vi "1.Main demo.vi"() -> ()   [LabVIEW 2010]
uses:
  UnderAutomation.Fanuc/UnderAutomation.Fanuc.lvlib
  C:/Users/fg/Documents/Fanuc.vi/LabVIEW_2024/UnderAutomation.Fanuc/lib/UnderAutomation.Fanuc.dll
  LabVIEW_2024/UnderAutomation.Fanuc/lib/UnderAutomation.Fanuc.dll
panel:
  out "SNPX connected":bool
  out "FTP connected":bool
  out "Telnet connected":bool
  in  "Tab Control":T1(tab)
  in  "Disconnect":bool
  in  "Test":bool
  in  "Key":string
  in  "Licensee":string
  in  "Use SNPX":bool
  in  "FTP password":string
  in  "FTP user":string
  in  "Use FTP":bool
  in  "Connect":bool
  in  "Telnet password":string
  in  "Use Telnet":bool
  in  "ConnectRoboguide":bool
  in  "RoboguideRobotPath":path caption="Path to \"Robot\" ROBOGUIDE folder that contains services.txt"
  in  "IP":string caption="Robot IP Address"
  out "License state":string
  out "Connect error":string
  in  "Unsimulate all":bool
  in  "Unsimulate":bool
  in  "Simulate":bool
  in  "Set port value":bool
  in  "Variable set value":bool
  in  "Variable new value":string caption="New value"
  in  "Variable get value":bool
  in  "Variable name":string
  out "Telnet warning":string
  out "Current position":T2
  in  "Get current position":bool
  in  "Reset alarms":bool
  in  "Get task info":bool
  in  "Task name":string caption="Task name (program without extension)"
  in  "Abort all programs":bool
  in  "Clear variable":bool
  in  "Clear Program":bool
  in  "Hold":bool
  in  "Continue":bool
  in  "Abort":bool
  in  "Pause":bool
  in  "Program name":string caption="Program name without extension"
  in  "Run":bool
  out "TelnetError":string caption="Error :"
  out "TelnetSucceed":bool caption="Succeeded"
  out "KclCommand":string caption="Last command :"
  out "TaskInfo":T3
  out "Variable value":string
  in  "port":i32(ring) items=["DIN", "DOUT", "RDO", "OPOUT", "TPOUT", "WDI", "WDO", "AIN", "AOUT", "GIN", "GOUT"]
  in  "index":i32
  in  "value":i32
  out "FTP warning":string
  out "PosReg":T4(array[cluster])
  out "StrReg":string[](array[string])
  in  "Tab Control IO state":T5(tab)
  out "UI":cluster{"Id":i32, "Name":string, "Value":bool}[](array[cluster])
  out "UO":cluster{"Id":i32, "Name":string, "Value":bool}[](array[cluster])
  out "SI":cluster{"Id":i32, "Name":string, "Value":bool}[](array[cluster])
  out "SO":cluster{"Id":i32, "Name":string, "Value":bool}[](array[cluster])
  out "DIN":cluster{"Id":i32, "Name":string, "Value":bool}[](array[cluster])
  out "DOUT":cluster{"Id":i32, "Name":string, "Value":bool}[](array[cluster])
  out "RI":cluster{"Id":i32, "Name":string, "Value":bool}[](array[cluster])
  out "RO":cluster{"Id":i32, "Name":string, "Value":bool}[](array[cluster])
  out "FLG":cluster{"Id":i32, "Name":string, "Value":bool}[](array[cluster])
  in  "Tab Control position":enum32{"World", "Joints", "User frames"}(tab)
  out "World Positions":T6(array[cluster])
  out "JointsPosition":dbl[](array[numeric])
  out "UserFramePositions":T7(array[cluster])
  in  "Get current position":bool
  in  "Get IO State":bool
  in  "Port":i32(ring) items=["DIN", "DOUT", "UI", "UO", "SI", "SO", "RI", "RO", "FLG"]
  out "Errors":T8(array[cluster])
  in  "Get all errors":bool
  in  "Get safety status":bool
  out "SafetyStatus":T9
  out "NumReg":dbl[](array[numeric])
  in  "Get numeric registers":bool
  in  "Get string registers":bool
  in  "Get position registers":bool
  out "SNPX warning":string
  in  "Tab Control snpx register":enum32{"Cartesian", "Joints"}(tab)
  in  "Cartesian position 2":T10
  in  "Write cartesian position register":bool
  in  "Joints position":dbl[](array[numeric])
  in  "Write joints position register":bool
  in  "Position register":i32
  in  "Read position register":bool
  out "Value":string
  in  "New value":string
  in  "String register":i32
  in  "Read string register":bool
  in  "Write string register":bool
  in  "Continuous read world position":bool
  out "JointsPosition":dbl[](array[numeric])
  out "Cartesian position":T11
  out "UserTool":i16
  out "error out":errorcluster
  in  "Continuous read user frame position":bool
  in  "userFrame":i32
  out "Cartesian position":T11
  out "UserTool":i16
  out "error out 2":errorcluster
  in  "Numeric register":i32
  in  "New value":sgl
  out "Value":sgl
  in  "Read numeric register":bool
  in  "Write numeric register":bool
  out "UserFrame":i16
  out "UserTool":i16
  in  "stop":bool
  out "Snpx":refnum<k24>
  out "Ftp":refnum<k24>
  out "Telnet":refnum<k24>
  out "robot":refnum<k24>
  # "UnderAutomation"
  # "https://underautomation.com/fanuc"
  # "+"
  # "LabVIEW demo app for remote control and monitoring of your Fanuc robot"
  # "Connect to robot"
  # "2. Ensure you have a trial or lifetime valid license"
  # "1. Set Fanuc robot address"
  # "This is a commercial library, you have a 30-day trial period. But you can use it forever if you buy a perpetual licence for your company (regardless of the number of robot, applications or developers)."
  # "Connect to real robot"
  # "Connect to ROBOGUIDE"
  # "If you have a license :"
  # "3. Select the services you want to connect to"
  # "Telnet"
  # "FTP"
  # "SNPX"
  # "You need option R553 \"HMI Device SNPX\" or R651 FRL"
  # "How to enable Telnet : https://underautomation.com/fanuc/documentation/enable-telnet"
  # "See : https://underautomation.com/fanuc/documentation/snpx"
  # "4. Connect to the robot"
  # "Telnet"
  # "Variables"
  # "Program execution"
  # "Task"
  # "Ports"
  # "Current position"
  # "Alarms"
  # "FTP"
  # "Current Position"
  # "IO State"
  # "Errors"
  # "Registers"
  # "Safety status"
  # "SNPX"
  # "Numeric registers"
  # "String registers"
  # "Read world position"
  # "Read user frame position"
  # "Position registers"
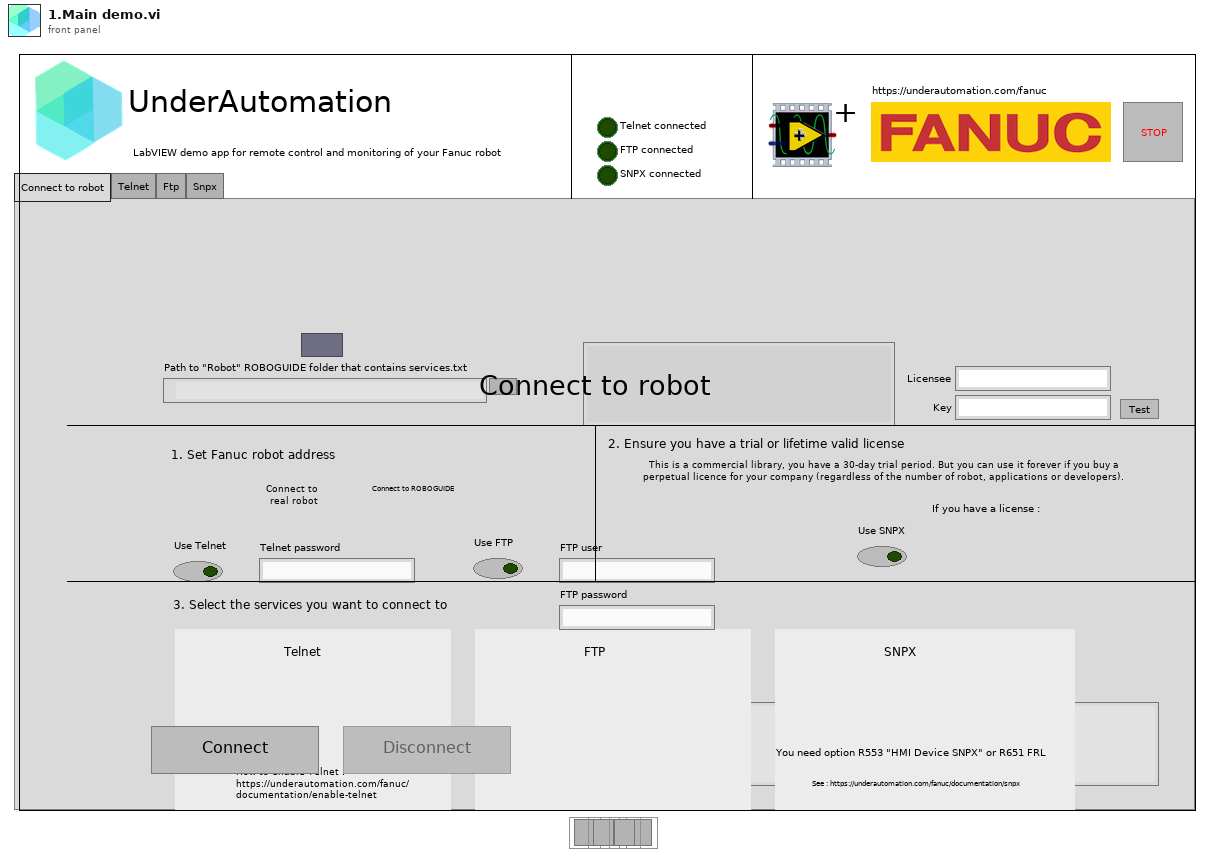
[diagram p1: front panel]
types:
  T1 = enum32{"Connect to robot", "Telnet", "Ftp", "Snpx"}
  T2 = cluster{"X":dbl, "Y":dbl, "Z":dbl, "W":dbl, "P":dbl, "R":dbl}
  T3 = cluster{"CurrentLine":i32, "RoutineName":string, "SystemTask":bool, "TaskName":string, "TaskNumber":i32, "TaskStatus":i32, "TaskStatusStr":string}
  T4 = cluster{"X":dbl, "Y":dbl, "Z":dbl, "W":dbl, "R":dbl, "P":dbl}[][]
  T5 = enum32{"UI", "UO", "SI", "SO", "DIN", "DOUT", "RI", "RO", "FLG"}
  T6 = cluster{"Tool":i32, "Cartesian position":cluster{cluster{"ArmFrontBack":i32, "ArmLeftRight":i32, "ArmUpDown":i32, "TurnAxis1":i32, "TurnAxis2":i32, "TurnAxis3":i32, "WristFlip":i32}, "X":dbl, "Y":dbl, "Z":dbl, "W":dbl, "P":dbl, "R":dbl}}[]
  T7 = cluster{"Frame":i32, "Tool":i32, "Cartesian position":cluster{cluster{"ArmFrontBack":i32, "ArmLeftRight":i32, "ArmUpDown":i32, "TurnAxis1":i32, "TurnAxis2":i32, "TurnAxis3":i32, "WristFlip":i32}, "X":dbl, "Y":dbl, "Z":dbl, "W":dbl, "P":dbl, "R":dbl}}[]
  T8 = cluster{"Id":i32, "IsReset":bool, "Text":string}[]
  T9 = cluster{"BeltBroken":bool, "ExternalEStop":bool, "FenceOpen":bool, "HandBroken":bool, "LowAirAlarm":bool, "NonTeacherEnb":bool, "OverTravel":bool, "SOPEStop":bool, "SVOFFDetect":bool, "TPDeadman":bool, "TPEnable":bool, "TPEStop":bool}
  T10 = cluster{"Configuration":cluster{"ArmFrontBack":i32, "ArmLeftRight":i32, "ArmUpDown":i32, "TurnAxis1":i32, "TurnAxis2":i32, "TurnAxis3":i32, "WristFlip":i32}, "X":dbl, "Y":dbl, "Z":dbl, "W":dbl, "P":dbl, "R":dbl}
  T11 = cluster{"Cartesian position":cluster{cluster{"ArmFrontBack":i32, "ArmLeftRight":i32, "ArmUpDown":i32, "TurnAxis1":i32, "TurnAxis2":i32, "TurnAxis3":i32, "WristFlip":i32}, "X":dbl, "Y":dbl, "Z":dbl, "W":dbl, "P":dbl, "R":dbl}, "Extension":cluster{"E1":dbl, "E2":dbl, "E3":dbl, "T4":i16, "T5":i16, "T6":i16}}
  T12 = enum8{"Enabled", "Disabled", "Disabled and Grayed Out"}
  T13 = cluster{"X":dbl, "Y":dbl, "Z":dbl, "W":dbl, "P":dbl, "R":dbl}[][]
  T14 = cluster{"Id":i32, "Values":dbl[], "UserFramePositions":cluster{"Frame":i32, "Tool":i32, "Cartesian position":cluster{cluster{"ArmFrontBack":i32, "ArmLeftRight":i32, "ArmUpDown":i32, "TurnAxis1":i32, "TurnAxis2":i32, "TurnAxis3":i32, "WristFlip":i32}, "X":dbl, "Y":dbl, "Z":dbl, "W":dbl, "P":dbl, "R":dbl}}[], "World Positions":cluster{"Tool":i32, "Cartesian position":cluster{cluster{"ArmFrontBack":i32, "ArmLeftRight":i32, "ArmUpDown":i32, "TurnAxis1":i32, "TurnAxis2":i32, "TurnAxis3":i32, "WristFlip":i32}, "X":dbl, "Y":dbl, "Z":dbl, "W":dbl, "P":dbl, "R":dbl}}[]}[]
  T15 = cluster{"Id":i32, "Name":string, "Port":i32, "Value":bool, "PortStr":string}[]
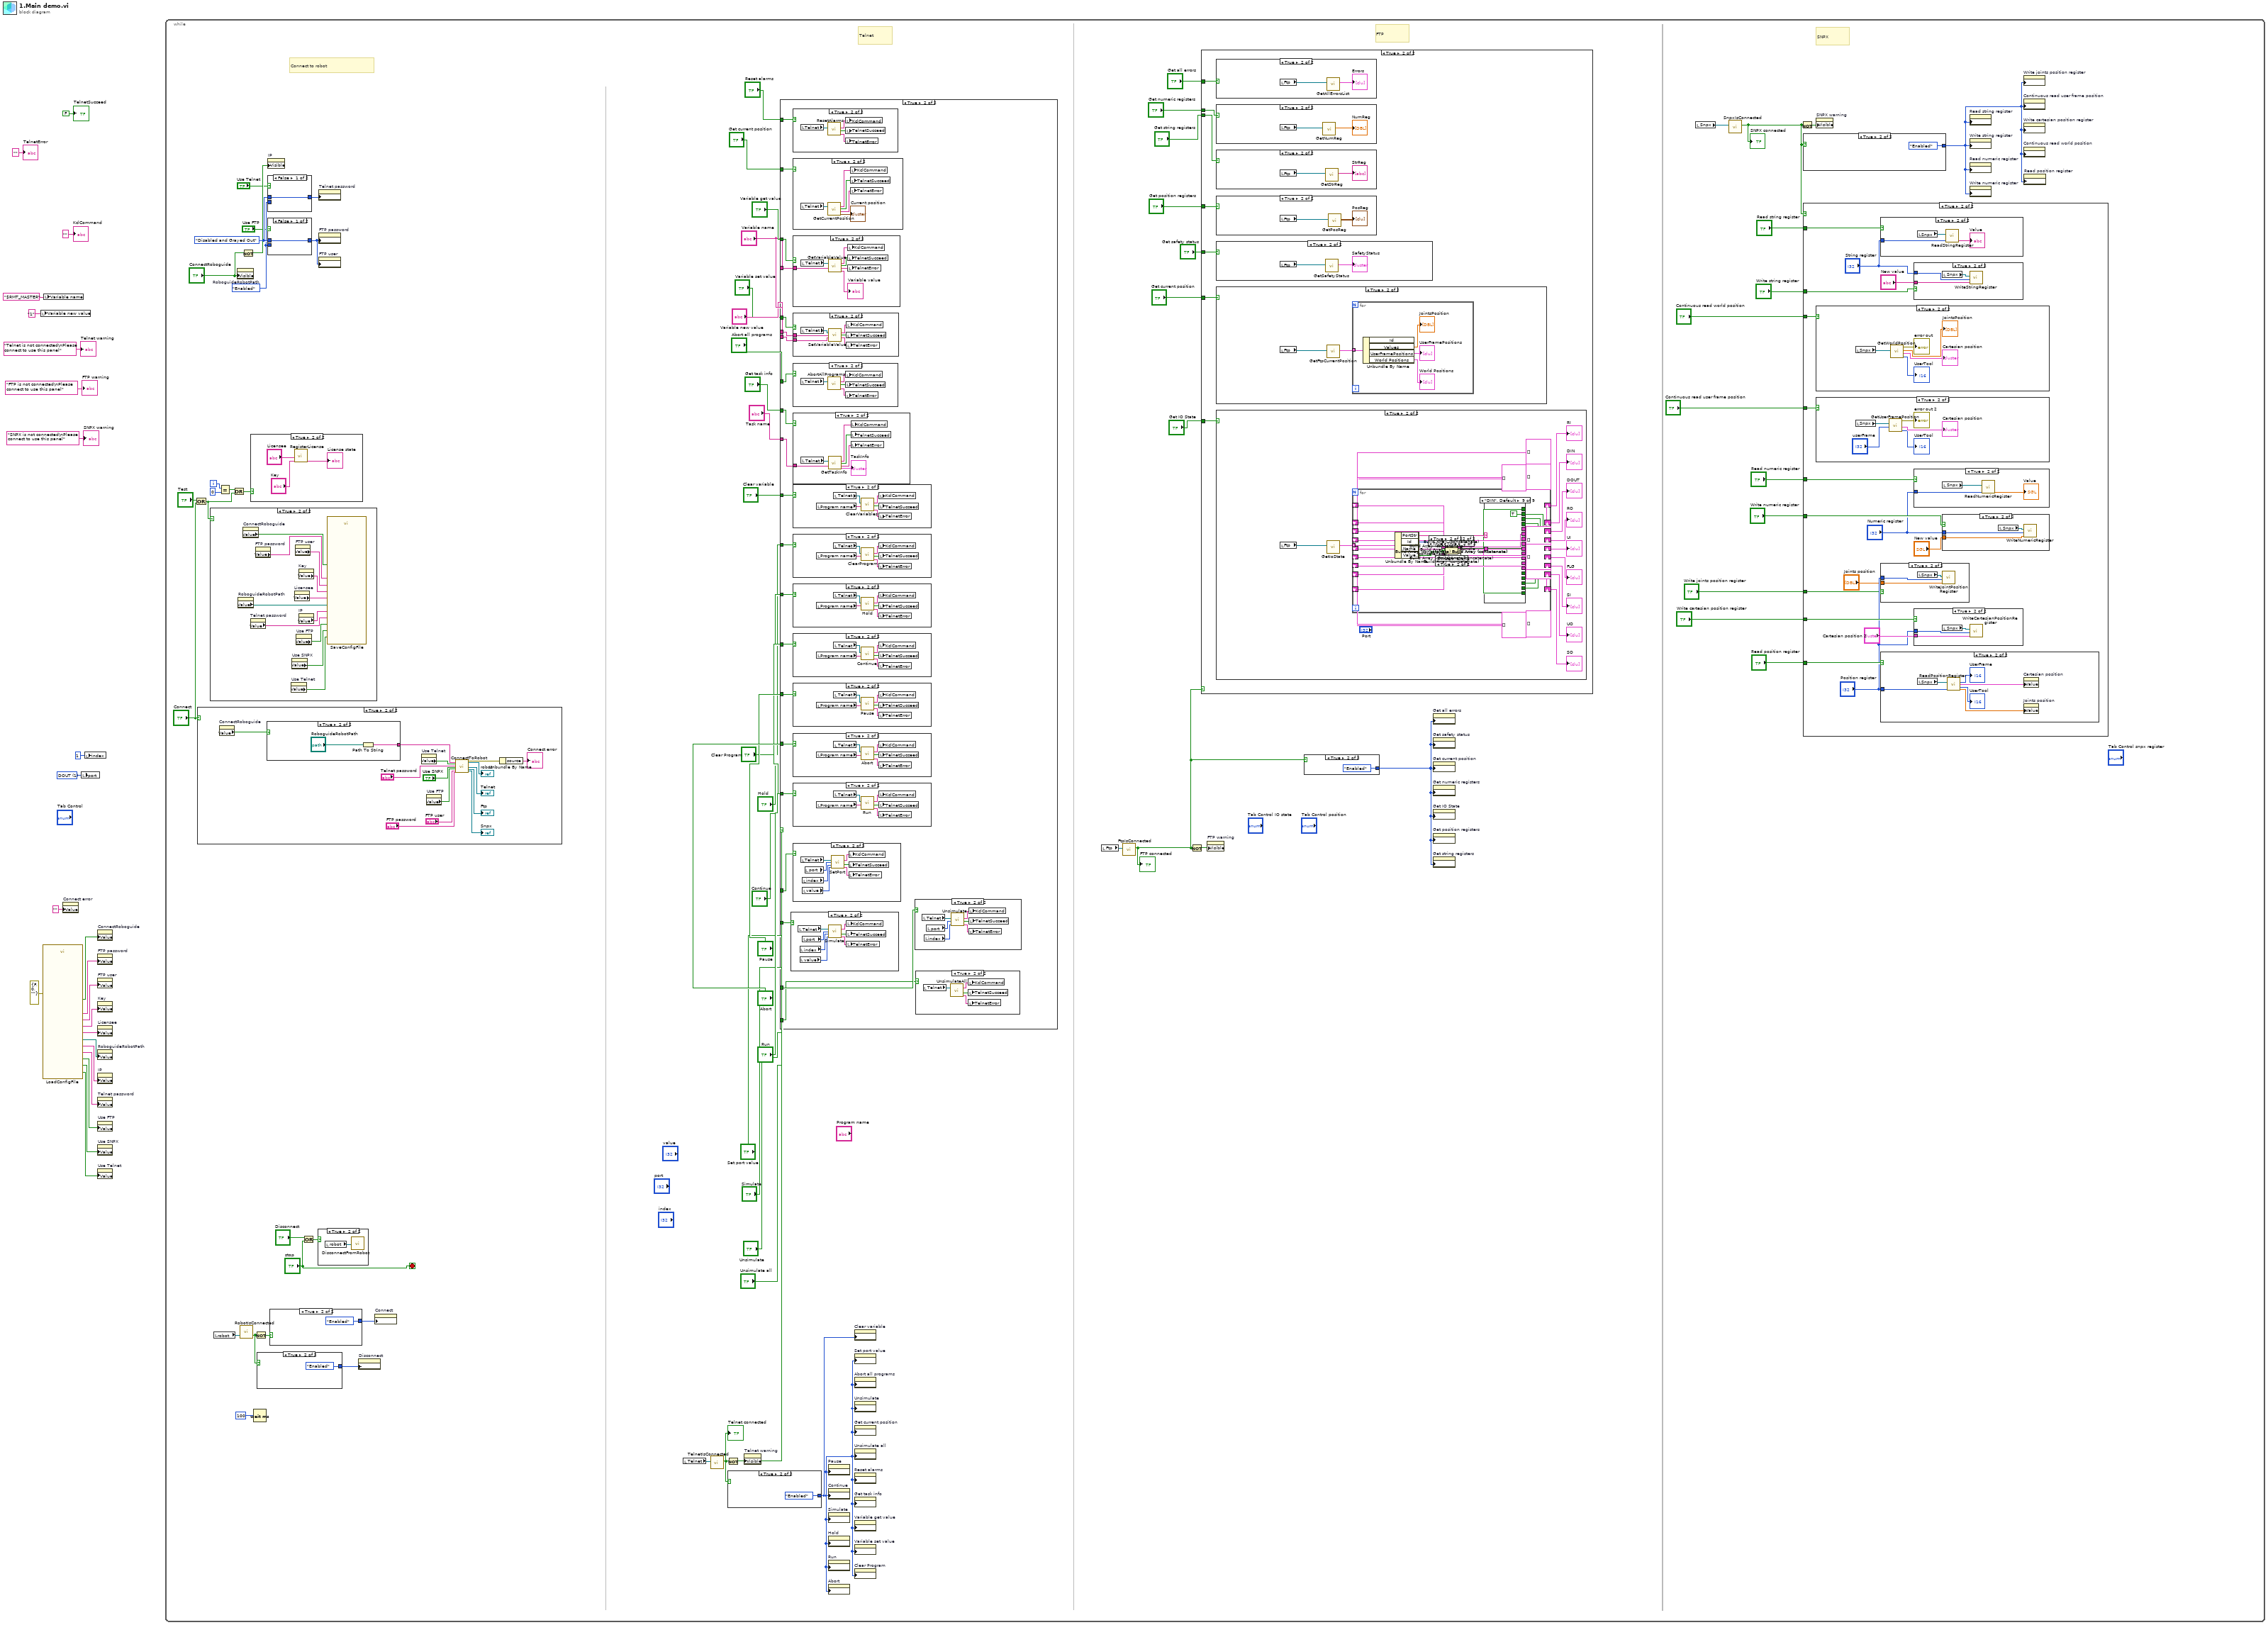
[diagram p0: block diagram]
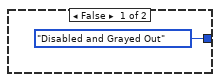
[diagram p2: hidden frame]
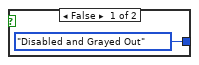
[diagram p13: hidden frame]
diagram:
  w3 = 1 items=["DIN", "DOUT", "RDO", "OPOUT", "TPOUT", "WDI", "WDO", "AIN", "AOUT", "GIN", "GOUT"] ("port")
  n1 = local write "Variable new value"("1" ("Variable new value")) -> ()
  n2 = call "LoadConfigFile.vi"("error in (no error)"=errorcluster {"status"=FALSE, "code"=0, "source"=""}) -> ("FTP password"=w20:string, "Licensee"=w12:string, "FTP user"=w19:string, "Key"=w13:string, "Use FTP"=w16:bool, "IP"=w22:string, "RoboguideRobotPath"=w18:path, "ConnectRoboguide"=w21:bool, "Use Telnet"=w14:bool, "Telnet password"=w17:string, "Use SNPX"=w15:bool)  [unwired: 15 in, 1 out]
  n3 = local write "Variable name"("$RMT_MASTER" ("Variable name")) -> ()
  n4 = property on="Connect error" class="Str"("Value"="" ("Connect error")) -> ()  [unwired: 2 in, 2 out]
  n5 = local write "port"(w3) -> ()
  n6 = local write "index"(1 ("index")) -> ()
  n7 = property on="ConnectRoboguide" class="Bool (strict)"("Value"=w21) -> ()  [unwired: 2 in, 2 out]
  n8 = property on="FTP password" class="Str"("Value"=w20) -> ()  [unwired: 2 in, 2 out]
  n9 = property on="FTP user" class="Str"("Value"=w19) -> ()  [unwired: 2 in, 2 out]
  n10 = property on="Key" class="Str"("Value"=w13) -> ()  [unwired: 2 in, 2 out]
  n11 = property on="Licensee" class="Str"("Value"=w12) -> ()  [unwired: 2 in, 2 out]
  n12 = property on="RoboguideRobotPath" class="Path"("Value"=w18) -> ()  [unwired: 2 in, 2 out]
  n13 = property on="IP" class="Str"("Value"=w22) -> ()  [unwired: 2 in, 2 out]
  n14 = property on="Telnet password" class="Str"("Value"=w17) -> ()  [unwired: 2 in, 2 out]
  n15 = property on="Use FTP" class="Bool (strict)"("Value"=w16) -> ()  [unwired: 2 in, 2 out]
  n16 = property on="Use SNPX" class="Bool (strict)"("Value"=w15) -> ()  [unwired: 2 in, 2 out]
  n17 = property on="Use Telnet" class="Bool (strict)"("Value"=w14) -> ()  [unwired: 2 in, 2 out]
  n18 = while {
    i -> [w90]
    stop <- "stop" stop-if-true
    w82 = T12."Enabled" ("Disabled")
    w83 = T12."Disabled and Grayed Out" ("Disabled")
    # "SNPX"
    # "FTP"
    # "Telnet"
    # "Connect to robot"
    n19 = Or(x="Test", y="Connect") -> (x .or. y?=w87:bool)
    n20 = case shown="True" "Connect" {
      frame False {
      }
      frame True {
        n21 = property on="ConnectRoboguide" class="Bool (strict)"() -> ("Value"=w438:bool)  [unwired: 2 in, 2 out]
        n22 = case shown="True" w438 {
          tunnel: ["IP" w440] -> w437
          frame False {
          }
          frame True {
            n23 = Path To String(path="RoboguideRobotPath") -> (string=w440:string)
          }
        }
        n24 = property on="Use Telnet" class="Bool (strict)"() -> ("Value"=w433:bool)  [unwired: 2 in, 2 out]
        n25 = property on="Use FTP" class="Bool (strict)"() -> ("Value"=w432:bool)  [unwired: 2 in, 2 out]
        n26 = call "ConnectToRobot.vi"("address"=w437, "Telnet enable"=w433, "Telnet KCL password"="Telnet password", "SNPX enable"="Use SNPX", "FTP enable"=w432, "FTP user"="FTP user", "FTP password"="FTP password") -> ("error out"=w431:errorcluster, "robot"=→"robot":refnum<k24>, "Telnet"=→"Telnet":refnum<k24>, "Ftp"=→"Ftp":refnum<k24>, "Snpx"=→"Snpx":refnum<k24>)  [unwired: 16 in]
        n27 = Unbundle By Name(w431) -> ("source"=→"Connect error":string)
      }
    }
    n28 = case shown="True" w87 {
      frame False {
      }
      frame True {
        n29 = property on="RoboguideRobotPath" class="Path"() -> ("Value"=w419:path)  [unwired: 2 in, 2 out]
        n30 = property on="ConnectRoboguide" class="Bool (strict)"() -> ("Value"=w424:bool)  [unwired: 2 in, 2 out]
        n31 = property on="Telnet password" class="Str"() -> ("Value"=w417:string)  [unwired: 2 in, 2 out]
        n32 = property on="FTP password" class="Str"() -> ("Value"=w423:string)  [unwired: 2 in, 2 out]
        n33 = property on="Use Telnet" class="Bool (strict)"() -> ("Value"=w414:bool)  [unwired: 2 in, 2 out]
        n34 = property on="Use SNPX" class="Bool (strict)"() -> ("Value"=w415:bool)  [unwired: 2 in, 2 out]
        n35 = property on="Licensee" class="Str"() -> ("Value"=w420:string)  [unwired: 2 in, 2 out]
        n36 = property on="FTP user" class="Str"() -> ("Value"=w422:string)  [unwired: 2 in, 2 out]
        n37 = property on="Use FTP" class="Bool (strict)"() -> ("Value"=w416:bool)  [unwired: 2 in, 2 out]
        n38 = property on="Key" class="Str"() -> ("Value"=w421:string)  [unwired: 2 in, 2 out]
        n39 = property on="IP" class="Str"() -> ("Value"=w418:string)  [unwired: 2 in, 2 out]
        n40 = call "SaveConfigFile.vi"("IP"=w418, "RoboguideRobotPath"=w419, "ConnectRoboguide"=w424, "Use Telnet"=w414, "Telnet password"=w417, "Use FTP"=w416, "FTP user"=w422, "FTP password"=w423, "Use SNPX"=w415, "Licensee"=w420, "Key"=w421) -> ()  [unwired: 17 in]
      }
    }
    n41 = local read "robot"() -> (w57:refnum<k24>)
    n42 = Equal?(x=w90, y=0) -> (x = y?=w88:bool)
    n43 = Or(x=w88, y=w87) -> (x .or. y?=w86:bool)
    n44 = property on="RoboguideRobotPath" class="Path"("Visible"="ConnectRoboguide") -> ()  [unwired: 2 in, 2 out]
    n45 = call "RobotIsConnected.vi"("robot"=w57) -> ("Connected"=w55:bool)  [unwired: 1 in, 1 out]
    n46 = Not(x="ConnectRoboguide") -> (.not. x?=w94:bool)
    n47 = case shown="True" w86 {
      frame False {
      }
      frame True {
        n48 = call "RegisterLicense.vi"("key"="Key", "licensee"="Licensee") -> ("status"=→"License state":string)  [unwired: 7 in, 2 out]
      }
    }
    n49 = Wait (ms)(milliseconds to wait=u32 100) -> ()  [unwired: 1 out]
    n50 = Not(x=w55) -> (.not. x?=w56:bool)
    n51 = case shown="True" w55 {
      tunnel: [T12."Disabled and Grayed Out" ("Disabled") T12."Enabled" ("Disabled")] -> w54
      frame False {
      }
      frame True {
      }
    }
    n52 = property on="IP" class="Str"("Visible"=w94) -> ()  [unwired: 2 in, 2 out]
    n53 = case shown="False" "Use Telnet" {
      tunnel: w82 -> [_ w410]
      tunnel: [w409 w410] -> w84
      tunnel: w83 -> [w409 _]
      frame False {
      }
      frame True {
      }
    }
    n54 = case shown="False" "Use FTP" {
      tunnel: w82 -> [_ w408]
      tunnel: [w407 w408] -> w80
      tunnel: w83 -> [w407 _]
      frame False {
      }
      frame True {
      }
    }
    n55 = case shown="True" w56 {
      tunnel: [T12."Disabled and Grayed Out" ("Disabled") T12."Enabled" ("Disabled")] -> w53
      frame False {
      }
      frame True {
      }
    }
    n56 = Or(x="Disconnect", y="stop") -> (x .or. y?=w59:bool)
    n57 = case shown="True" w59 {
      frame False {
      }
      frame True {
        n58 = local read "robot"() -> (w293:refnum<k24>)
        n59 = call "DisconnectFromRobot.vi"("robot"=w293) -> ()  [unwired: 26 in, 1 out]
      }
    }
    n60 = property on="Telnet password" class="Str"("DisabledEnum"=w84) -> ()  [unwired: 2 in, 2 out]
    n61 = property on="FTP password" class="Str"("DisabledEnum"=w80) -> ()  [unwired: 2 in, 2 out]
    n62 = property on="FTP user" class="Str"("DisabledEnum"=w80) -> ()  [unwired: 2 in, 2 out]
    n63 = property on="Disconnect" class="Bool"("DisabledEnum"=w54) -> ()  [unwired: 2 in, 2 out]
    n64 = property on="Connect" class="Bool"("DisabledEnum"=w53) -> ()  [unwired: 2 in, 2 out]
    n65 = local read "Telnet"() -> (w79:refnum<k24>)
    n66 = call "TelnetIsConnected.vi"("Telnet"=w79) -> ("Connected"=w77:bool)  [unwired: 9 in, 1 out]
    "Telnet connected" <- w77
    n67 = Not(x=w77) -> (.not. x?=w76:bool)
    n68 = case shown="True" w77 {
      tunnel: [T12."Disabled and Grayed Out" ("Disabled") T12."Enabled" ("Disabled")] -> w48
      frame False {
      }
      frame True {
      }
    }
    n69 = property on="Telnet warning" class="Str"("Visible"=w76) -> ()  [unwired: 2 in, 2 out]
    n70 = case shown="True" w77 {
      tunnel: "Run" -> [_ w316]
      tunnel: "Abort" -> [_ w315]
      tunnel: "Pause" -> [_ w314]
      tunnel: "Continue" -> [_ w313]
      tunnel: "Hold" -> [_ w312]
      tunnel: "Clear variable" -> [_ w311]
      tunnel: "Clear Program" -> [_ w310]
      tunnel: "Abort all programs" -> [_ w309]
      tunnel: "Task name" -> [_ w308]
      tunnel: "Get task info" -> [_ w307]
      tunnel: "Reset alarms" -> [_ w306]
      tunnel: "Get current position" -> [_ w305]
      tunnel: "Variable get value" -> [_ w304]
      tunnel: "Variable name" -> [_ w303]
      tunnel: "Variable name" -> [_ w302]
      tunnel: "Variable new value" -> [_ w301]
      tunnel: "Variable set value" -> [_ w300]
      tunnel: "Set port value" -> [_ w299]
      tunnel: "Simulate" -> [_ w298]
      tunnel: "Unsimulate" -> [_ w297]
      tunnel: "Unsimulate all" -> [_ w296]
      frame False {
      }
      frame True {
        n71 = case shown="True" w298 {
          frame False {
          }
          frame True {
            n72 = local read "Telnet"() -> (w330:refnum<k24>)
            n73 = local read "index"() -> (w327:i32)
            n74 = local read "value"() -> (w329:i32)
            n75 = local read "port"() -> (w328:i32)
            n76 = call "Simulate.vi"("Telnet"=w330, "port"=w328, "index"=w327, "value"=w329) -> ("KclCommand"=w333:string, "Succeed"=w332:bool, "ErrorText"=w331:string)  [unwired: 8 in, 1 out]
            n77 = local write "KclCommand"(w333) -> ()
            n78 = local write "TelnetSucceed"(w332) -> ()
            n79 = local write "TelnetError"(w331) -> ()
          }
        }
        n80 = case shown="True" w306 {
          frame False {
          }
          frame True {
            n81 = local read "Telnet"() -> (w361:refnum<k24>)
            n82 = call "ResetAlarms.vi"("Telnet"=w361) -> ("ErrorText"=w359:string, "Succeed"=w360:bool, "KclCommand"=w358:string)  [unwired: 7 in, 1 out]
            n83 = local write "KclCommand"(w358) -> ()
            n84 = local write "TelnetSucceed"(w360) -> ()
            n85 = local write "TelnetError"(w359) -> ()
          }
        }
        n86 = case shown="True" w305 {
          frame False {
          }
          frame True {
            n87 = local read "Telnet"() -> (w357:refnum<k24>)
            n88 = call "GetCurrentPosition.vi"("Telnet"=w357) -> ("KclCommand"=w355:string, "Succeed"=w354:bool, "ErrorText"=w353:string, "Position"=→"Current position":T2)  [unwired: 10 in, 1 out]
            n89 = local write "KclCommand"(w355) -> ()
            n90 = local write "TelnetSucceed"(w354) -> ()
            n91 = local write "TelnetError"(w353) -> ()
          }
        }
        n92 = case shown="True" w304 {
          tunnel: w303 -> [_ w351]
          frame False {
          }
          frame True {
            n93 = local read "Telnet"() -> (w352:refnum<k24>)
            n94 = call "GetVariableValue.vi"("Telnet"=w352, "name"=w351) -> ("KclCommand"=w347:string, "Succeed"=w348:bool, "ErrorText"=w349:string, "RawValue"=→"Variable value":string)  [unwired: 9 in, 1 out]
            n95 = local write "KclCommand"(w347) -> ()
            n96 = local write "TelnetSucceed"(w348) -> ()
            n97 = local write "TelnetError"(w349) -> ()
          }
        }
        n98 = case shown="True" w300 {
          tunnel: w302 -> [_ w345]
          tunnel: w301 -> [_ w344]
          frame False {
          }
          frame True {
            n99 = local read "Telnet"() -> (w346:refnum<k24>)
            n100 = call "SetVariableValue.vi"("Telnet"=w346, "value"=w344, "name"=w345) -> ("KclCommand"=w343:string, "Succeed"=w342:bool, "ErrorText"=w341:string)  [unwired: 9 in, 1 out]
            n101 = local write "KclCommand"(w343) -> ()
            n102 = local write "TelnetSucceed"(w342) -> ()
            n103 = local write "TelnetError"(w341) -> ()
          }
        }
        n104 = case shown="True" w309 {
          frame False {
          }
          frame True {
            n105 = local read "Telnet"() -> (w368:refnum<k24>)
            n106 = call "AbortAllPrograms.vi"("Telnet"=w368) -> ("ErrorText"=w369:string, "Succeed"=w370:bool, "KclCommand"=w371:string)  [unwired: 7 in, 1 out]
            n107 = local write "KclCommand"(w371) -> ()
            n108 = local write "TelnetSucceed"(w370) -> ()
            n109 = local write "TelnetError"(w369) -> ()
          }
        }
        n110 = case shown="True" w307 {
          tunnel: w308 -> [_ w366]
          frame False {
          }
          frame True {
            n111 = local read "Telnet"() -> (w367:refnum<k24>)
            n112 = call "GetTaskInfo.vi"("Telnet"=w367, "task"=w366) -> ("KclCommand"=w364:string, "Succeed"=w363:bool, "ErrorText"=w362:string, "TaskInfo"=→"TaskInfo":T3)  [unwired: 9 in, 1 out]
            n113 = local write "KclCommand"(w364) -> ()
            n114 = local write "TelnetSucceed"(w363) -> ()
            n115 = local write "TelnetError"(w362) -> ()
          }
        }
        n116 = case shown="True" w311 {
          frame False {
          }
          frame True {
            n117 = local read "Program name"() -> (w372:string)
            n118 = local read "Telnet"() -> (w373:refnum<k24>)
            n119 = call "ClearVariables.vi"("program"=w372, "Telnet"=w373) -> ("ErrorText"=w374:string, "Succeed"=w375:bool, "KclCommand"=w376:string)  [unwired: 6 in, 1 out]
            n120 = local write "KclCommand"(w376) -> ()
            n121 = local write "TelnetSucceed"(w375) -> ()
            n122 = local write "TelnetError"(w374) -> ()
          }
        }
        n123 = case shown="True" w310 {
          frame False {
          }
          frame True {
            n124 = local read "Program name"() -> (w377:string)
            n125 = local read "Telnet"() -> (w378:refnum<k24>)
            n126 = call "ClearProgram.vi"("program"=w377, "Telnet"=w378) -> ("ErrorText"=w379:string, "Succeed"=w380:bool, "KclCommand"=w381:string)  [unwired: 6 in, 1 out]
            n127 = local write "KclCommand"(w381) -> ()
            n128 = local write "TelnetSucceed"(w380) -> ()
            n129 = local write "TelnetError"(w379) -> ()
          }
        }
        n130 = case shown="True" w312 {
          frame False {
          }
          frame True {
            n131 = local read "Program name"() -> (w382:string)
            n132 = local read "Telnet"() -> (w383:refnum<k24>)
            n133 = call "Hold.vi"("program"=w382, "Telnet"=w383) -> ("ErrorText"=w384:string, "Succeed"=w385:bool, "KclCommand"=w386:string)  [unwired: 6 in, 1 out]
            n134 = local write "KclCommand"(w386) -> ()
            n135 = local write "TelnetSucceed"(w385) -> ()
            n136 = local write "TelnetError"(w384) -> ()
          }
        }
        n137 = case shown="True" w313 {
          frame False {
          }
          frame True {
            n138 = local read "Program name"() -> (w387:string)
            n139 = local read "Telnet"() -> (w388:refnum<k24>)
            n140 = call "Continue.vi"("program"=w387, "Telnet"=w388) -> ("ErrorText"=w389:string, "Succeed"=w390:bool, "KclCommand"=w391:string)  [unwired: 6 in, 1 out]
            n141 = local write "KclCommand"(w391) -> ()
            n142 = local write "TelnetSucceed"(w390) -> ()
            n143 = local write "TelnetError"(w389) -> ()
          }
        }
        n144 = case shown="True" w314 {
          frame False {
          }
          frame True {
            n145 = local read "Program name"() -> (w392:string)
            n146 = local read "Telnet"() -> (w393:refnum<k24>)
            n147 = call "Pause.vi"("program"=w392, "Telnet"=w393) -> ("ErrorText"=w394:string, "Succeed"=w395:bool, "KclCommand"=w396:string)  [unwired: 6 in, 1 out]
            n148 = local write "KclCommand"(w396) -> ()
            n149 = local write "TelnetSucceed"(w395) -> ()
            n150 = local write "TelnetError"(w394) -> ()
          }
        }
        n151 = case shown="True" w315 {
          frame False {
          }
          frame True {
            n152 = local read "Program name"() -> (w397:string)
            n153 = local read "Telnet"() -> (w398:refnum<k24>)
            n154 = call "Abort.vi"("program"=w397, "Telnet"=w398) -> ("ErrorText"=w399:string, "Succeed"=w400:bool, "KclCommand"=w401:string)  [unwired: 6 in, 1 out]
            n155 = local write "KclCommand"(w401) -> ()
            n156 = local write "TelnetSucceed"(w400) -> ()
            n157 = local write "TelnetError"(w399) -> ()
          }
        }
        n158 = case shown="True" w316 {
          frame False {
          }
          frame True {
            n159 = local read "Program name"() -> (w402:string)
            n160 = local read "Telnet"() -> (w403:refnum<k24>)
            n161 = call "Run.vi"("program"=w402, "Telnet"=w403) -> ("ErrorText"=w404:string, "Succeed"=w405:bool, "KclCommand"=w406:string)  [unwired: 6 in, 1 out]
            n162 = local write "KclCommand"(w406) -> ()
            n163 = local write "TelnetSucceed"(w405) -> ()
            n164 = local write "TelnetError"(w404) -> ()
          }
        }
        n165 = case shown="True" w299 {
          frame False {
          }
          frame True {
            n166 = local read "Telnet"() -> (w337:refnum<k24>)
            n167 = local read "index"() -> (w334:i32)
            n168 = local read "value"() -> (w336:i32)
            n169 = local read "port"() -> (w335:i32)
            n170 = call "SetPort.vi"("Telnet"=w337, "port"=w335, "index"=w334, "value"=w336) -> ("KclCommand"=w340:string, "Succeed"=w339:bool, "ErrorText"=w338:string)  [unwired: 8 in, 1 out]
            n171 = local write "KclCommand"(w340) -> ()
            n172 = local write "TelnetSucceed"(w339) -> ()
            n173 = local write "TelnetError"(w338) -> ()
          }
        }
        n174 = case shown="True" w297 {
          frame False {
          }
          frame True {
            n175 = local read "Telnet"() -> (w323:refnum<k24>)
            n176 = local read "index"() -> (w321:i32)
            n177 = local read "port"() -> (w322:i32)
            n178 = call "Unsimulate.vi"("index"=w321, "port"=w322, "Telnet"=w323) -> ("ErrorText"=w324:string, "Succeed"=w325:bool, "KclCommand"=w326:string)  [unwired: 5 in, 1 out]
            n179 = local write "KclCommand"(w326) -> ()
            n180 = local write "TelnetSucceed"(w325) -> ()
            n181 = local write "TelnetError"(w324) -> ()
          }
        }
        n182 = case shown="True" w296 {
          frame False {
          }
          frame True {
            n183 = local read "Telnet"() -> (w317:refnum<k24>)
            n184 = call "UnsimulateAll.vi"("Telnet"=w317) -> ("KclCommand"=w320:string, "Succeed"=w319:bool, "ErrorText"=w318:string)  [unwired: 11 in, 1 out]
            n185 = local write "KclCommand"(w320) -> ()
            n186 = local write "TelnetSucceed"(w319) -> ()
            n187 = local write "TelnetError"(w318) -> ()
          }
        }
      }
    }
    n188 = property on="Pause" class="Bool"("DisabledEnum"=w48) -> ()  [unwired: 2 in, 2 out]
    n189 = property on="Continue" class="Bool"("DisabledEnum"=w48) -> ()  [unwired: 2 in, 2 out]
    n190 = property on="Simulate" class="Bool"("DisabledEnum"=w48) -> ()  [unwired: 2 in, 2 out]
    n191 = property on="Hold" class="Bool"("DisabledEnum"=w48) -> ()  [unwired: 2 in, 2 out]
    n192 = property on="Run" class="Bool"("DisabledEnum"=w48) -> ()  [unwired: 2 in, 2 out]
    n193 = property on="Abort" class="Bool"("DisabledEnum"=w48) -> ()  [unwired: 2 in, 2 out]
    n194 = property on="Clear variable" class="Bool"("DisabledEnum"=w48) -> ()  [unwired: 2 in, 2 out]
    n195 = property on="Set port value" class="Bool"("DisabledEnum"=w48) -> ()  [unwired: 2 in, 2 out]
    n196 = property on="Abort all programs" class="Bool"("DisabledEnum"=w48) -> ()  [unwired: 2 in, 2 out]
    n197 = property on="Unsimulate" class="Bool"("DisabledEnum"=w48) -> ()  [unwired: 2 in, 2 out]
    n198 = property on="Get current position" class="Bool"("DisabledEnum"=w48) -> ()  [unwired: 2 in, 2 out]
    n199 = property on="Unsimulate all" class="Bool"("DisabledEnum"=w48) -> ()  [unwired: 2 in, 2 out]
    n200 = property on="Reset alarms" class="Bool"("DisabledEnum"=w48) -> ()  [unwired: 2 in, 2 out]
    n201 = property on="Get task info" class="Bool"("DisabledEnum"=w48) -> ()  [unwired: 2 in, 2 out]
    n202 = property on="Variable get value" class="Bool"("DisabledEnum"=w48) -> ()  [unwired: 2 in, 2 out]
    n203 = property on="Variable set value" class="Bool"("DisabledEnum"=w48) -> ()  [unwired: 2 in, 2 out]
    n204 = property on="Clear Program" class="Bool"("DisabledEnum"=w48) -> ()  [unwired: 2 in, 2 out]
    n205 = local read "Ftp"() -> (w47:refnum<k24>)
    n206 = call "FtpIsConnected.vi"("Ftp"=w47) -> ("Connected"=w38:bool)  [unwired: 9 in, 1 out]
    "FTP connected" <- w38
    n207 = Not(x=w38) -> (.not. x?=w39:bool)
    n208 = case shown="True" w38 {
      tunnel: "Get current position" -> [_ w156]
      tunnel: "Get IO State" -> [_ w155]
      tunnel: "Get all errors" -> [_ w154]
      tunnel: "Get safety status" -> [_ w153]
      tunnel: "Get numeric registers" -> [_ w152]
      tunnel: "Get string registers" -> [_ w151]
      tunnel: "Get position registers" -> [_ w150]
      frame False {
      }
      frame True {
        n209 = case shown="True" w154 {
          frame False {
          }
          frame True {
            n210 = local read "Ftp"() -> (w166:refnum<k24>)
            n211 = call "GetAllErrorsList.vi"("Ftp"=w166) -> ("Errors"=→"Errors":T8)  [unwired: 9 in, 1 out]
          }
        }
        n212 = case shown="True" w152 {
          frame False {
          }
          frame True {
            n213 = local read "Ftp"() -> (w162:refnum<k24>)
            n214 = call "GetNumReg.vi"("Ftp"=w162) -> ("NumReg"=→"NumReg":dbl[])  [unwired: 9 in, 1 out]
          }
        }
        n215 = case shown="True" w151 {
          frame False {
          }
          frame True {
            n216 = local read "Ftp"() -> (w160:refnum<k24>)
            n217 = call "GetStrReg.vi"("Ftp"=w160) -> ("StrReg"=→"StrReg":string[])  [unwired: 9 in, 1 out]
          }
        }
        n218 = case shown="True" w150 {
          frame False {
          }
          frame True {
            n219 = local read "Ftp"() -> (w158:refnum<k24>)
            n220 = call "GetPosReg.vi"("Ftp"=w158) -> ("PosReg"=→"PosReg":T13)  [unwired: 9 in, 1 out]
          }
        }
        n221 = case shown="True" w153 {
          frame False {
          }
          frame True {
            n222 = local read "Ftp"() -> (w164:refnum<k24>)
            n223 = call "GetSafetyStatus.vi"("Ftp"=w164) -> ("SafetyStatus"=→"SafetyStatus":T9)  [unwired: 9 in, 1 out]
          }
        }
        n224 = case shown="True" w156 {
          frame False {
          }
          frame True {
            n225 = local read "Ftp"() -> (w284:refnum<k24>)
            n226 = call "GetFtpCurrentPosition.vi"("Ftp"=w284) -> ("Current position"=w283:T14)  [unwired: 9 in, 1 out]
            n227 = for {
              tunnel: w283 -> [w287] mode=indexing
              n228 = Unbundle By Name(w287) -> ("Values"=→"JointsPosition":dbl[], "UserFramePositions"=→"UserFramePositions":T7, "World Positions"=→"World Positions":T6)  [unwired: 1 out]
            }
          }
        }
        n229 = case shown="True" w155 {
          frame False {
          }
          frame True {
            n230 = local read "Ftp"() -> (w186:refnum<k24>)
            n231 = call "GetIoState.vi"("Ftp"=w186) -> ("IO States"=w185:T15)  [unwired: 9 in, 1 out]
            n232 = for {
              tunnel: w185 -> [w228] mode=indexing
              shift-right: [w203] -> w184
              shift-left: cluster{"Id":i32, "Name":string, "Value":bool}[] [] ("Array") -> [w204]
              shift-right: [w201] -> w183
              shift-left: cluster{"Id":i32, "Name":string, "Value":bool}[] [] ("Array") -> [w202]
              shift-right: [w199] -> w176
              shift-left: cluster{"Id":i32, "Name":string, "Value":bool}[] [] ("Array") -> [w200]
              shift-right: [w197] -> w182
              shift-left: cluster{"Id":i32, "Name":string, "Value":bool}[] [] ("Array") -> [w198]
              shift-right: [w195] -> w181
              shift-left: cluster{"Id":i32, "Name":string, "Value":bool}[] [] ("Array") -> [w196]
              shift-right: [w193] -> w180
              shift-left: cluster{"Id":i32, "Name":string, "Value":bool}[] [] ("Array") -> [w194]
              shift-right: [w191] -> w179
              shift-left: cluster{"Id":i32, "Name":string, "Value":bool}[] [] ("Array") -> [w192]
              shift-right: [w189] -> w178
              shift-left: cluster{"Id":i32, "Name":string, "Value":bool}[] [] ("Array") -> [w190]
              shift-right: [w187] -> w177
              shift-left: cluster{"Id":i32, "Name":string, "Value":bool}[] [] ("Array") -> [w188]
              n233 = Unbundle By Name(w228) -> ("PortStr"=w216:string, "Id"=w227:i32, "Name"=w226:string, "Value"=w225:bool)
              n234 = Bundle("Id"=w227, "Name"=w226, "Value"=w225) -> (w223:cluster{"Id":i32, "Name":string, "Value":bool})  [unwired: 1 in]
              n235 = case shown="\"DIN\", Default" w216 {
                tunnel: [_ _ _ _ _ _ _ w280 _] -> w224
                tunnel: w223 -> [w266 w268 w270 w272 w274 w276 w278 w280 w282]
                tunnel: [_ _ _ _ _ _ w278 _ _] -> w222
                tunnel: [_ _ _ _ _ _ _ _ w282] -> w214
                tunnel: [w266 _ _ _ _ _ _ _ _] -> w221
                tunnel: [_ w268 _ _ _ _ _ _ _] -> w220
                tunnel: [_ _ w270 _ _ _ _ _ _] -> w219
                tunnel: [_ _ _ w272 _ _ _ _ _] -> w218
                tunnel: [_ _ _ _ w274 _ _ _ _] -> w217
                tunnel: [_ _ _ _ _ w276 _ _ _] -> w215
                tunnel: [_ _ TRUE _ _ _ _ _ _] -> w213
                tunnel: [_ _ _ TRUE _ _ _ _ _] -> w212
                tunnel: [_ _ _ _ TRUE _ _ _ _] -> w211
                tunnel: [_ _ _ _ _ TRUE _ _ _] -> w210
                tunnel: [_ _ _ _ _ _ TRUE _ _] -> w209
                tunnel: [_ _ _ _ _ _ _ TRUE _] -> w208
                tunnel: [_ _ _ _ _ _ _ _ TRUE] -> w207
                tunnel: [TRUE _ _ _ _ _ _ _ _] -> w206
                tunnel: [_ TRUE _ _ _ _ _ _ _] -> w205
                frame "DOUT" {
                }
                frame "UI" {
                }
                frame "UO" {
                }
                frame "SI" {
                }
                frame "SO" {
                }
                frame "RI" {
                }
                frame "RO" {
                }
                frame "FLG" {
                }
                frame "DIN", Default {
                }
              }
              n236 = case shown="True" w210 {
                tunnel: w188 -> [w229 w231]
                tunnel: w215 -> [_ w230]
                tunnel: [w229 w232] -> w187
                frame False {
                }
                frame True {
                  n237 = Build Array (concatenate)(w231, w230) -> (w232:cluster{"Id":i32, "Name":string, "Value":bool}[])
                }
              }
              n238 = case shown="True" w211 {
                tunnel: w190 -> [w233 w235]
                tunnel: w217 -> [_ w234]
                tunnel: [w233 w236] -> w189
                frame False {
                }
                frame True {
                  n239 = Build Array (concatenate)(w235, w234) -> (w236:cluster{"Id":i32, "Name":string, "Value":bool}[])
                }
              }
              n240 = case shown="True" w212 {
                tunnel: w192 -> [w237 w239]
                tunnel: w218 -> [_ w238]
                tunnel: [w237 w240] -> w191
                frame False {
                }
                frame True {
                  n241 = Build Array (concatenate)(w239, w238) -> (w240:cluster{"Id":i32, "Name":string, "Value":bool}[])
                }
              }
              n242 = case shown="True" w213 {
                tunnel: w194 -> [w241 w243]
                tunnel: w219 -> [_ w242]
                tunnel: [w241 w244] -> w193
                frame False {
                }
                frame True {
                  n243 = Build Array (concatenate)(w243, w242) -> (w244:cluster{"Id":i32, "Name":string, "Value":bool}[])
                }
              }
              n244 = case shown="True" w205 {
                tunnel: w196 -> [w245 w247]
                tunnel: w220 -> [_ w246]
                tunnel: [w245 w248] -> w195
                frame False {
                }
                frame True {
                  n245 = Build Array (concatenate)(w247, w246) -> (w248:cluster{"Id":i32, "Name":string, "Value":bool}[])
                }
              }
              n246 = case shown="True" w206 {
                tunnel: w198 -> [w249 w251]
                tunnel: w221 -> [_ w250]
                tunnel: [w249 w252] -> w197
                frame False {
                }
                frame True {
                  n247 = Build Array (concatenate)(w251, w250) -> (w252:cluster{"Id":i32, "Name":string, "Value":bool}[])
                }
              }
              n248 = case shown="True" w207 {
                tunnel: w200 -> [w253 w255]
                tunnel: w214 -> [_ w254]
                tunnel: [w253 w256] -> w199
                frame False {
                }
                frame True {
                  n249 = Build Array (concatenate)(w255, w254) -> (w256:cluster{"Id":i32, "Name":string, "Value":bool}[])
                }
              }
              n250 = case shown="True" w209 {
                tunnel: w202 -> [w257 w259]
                tunnel: w222 -> [_ w258]
                tunnel: [w257 w260] -> w201
                frame False {
                }
                frame True {
                  n251 = Build Array (concatenate)(w259, w258) -> (w260:cluster{"Id":i32, "Name":string, "Value":bool}[])
                }
              }
              n252 = case shown="True" w208 {
                tunnel: w204 -> [w261 w263]
                tunnel: w224 -> [_ w262]
                tunnel: [w261 w264] -> w203
                frame False {
                }
                frame True {
                  n253 = Build Array (concatenate)(w263, w262) -> (w264:cluster{"Id":i32, "Name":string, "Value":bool}[])
                }
              }
            }
            "FLG" <- w184
            "RO" <- w183
            "DIN" <- w176
            "DOUT" <- w182
            "UI" <- w181
            "UO" <- w180
            "SI" <- w179
            "SO" <- w178
            "RI" <- w177
          }
        }
      }
    }
    n254 = property on="FTP warning" class="Str"("Visible"=w39) -> ()  [unwired: 2 in, 2 out]
    n255 = case shown="True" w38 {
      tunnel: [T12."Disabled and Grayed Out" ("Disabled") T12."Enabled" ("Disabled")] -> w37
      frame False {
      }
      frame True {
      }
    }
    n256 = property on="Get all errors" class="Bool"("DisabledEnum"=w37) -> ()  [unwired: 2 in, 2 out]
    n257 = property on="Get safety status" class="Bool"("DisabledEnum"=w37) -> ()  [unwired: 2 in, 2 out]
    n258 = property on="Get current position" class="Bool"("DisabledEnum"=w37) -> ()  [unwired: 2 in, 2 out]
    n259 = property on="Get numeric registers" class="Bool"("DisabledEnum"=w37) -> ()  [unwired: 2 in, 2 out]
    n260 = property on="Get IO State" class="Bool"("DisabledEnum"=w37) -> ()  [unwired: 2 in, 2 out]
    n261 = property on="Get position registers" class="Bool"("DisabledEnum"=w37) -> ()  [unwired: 2 in, 2 out]
    n262 = property on="Get string registers" class="Bool"("DisabledEnum"=w37) -> ()  [unwired: 2 in, 2 out]
    n263 = local read "Snpx"() -> (w35:refnum<k24>)
    n264 = call "SnpxIsConnected.vi"("Snpx"=w35) -> ("Connected"=w25:bool)  [unwired: 9 in, 1 out]
    "SNPX connected" <- w25
    n265 = Not(x=w25) -> (.not. x?=w36:bool)
    n266 = case shown="True" w25 {
      tunnel: [T12."Disabled and Grayed Out" ("Disabled") T12."Enabled" ("Disabled")] -> w24
      frame False {
      }
      frame True {
      }
    }
    n267 = case shown="True" w25 {
      tunnel: "Continuous read world position" -> [_ w113]
      tunnel: "Continuous read user frame position" -> [_ w112]
      tunnel: "Read numeric register" -> [_ w111]
      tunnel: "Write numeric register" -> [_ w110]
      tunnel: "Read string register" -> [_ w105]
      tunnel: "Write string register" -> [_ w104]
      tunnel: "Read position register" -> [_ w103]
      tunnel: "Write cartesian position register" -> [_ w102]
      tunnel: "Write joints position register" -> [_ w98]
      frame False {
      }
      frame True {
        n268 = case shown="True" w113 {
          frame False {
          }
          frame True {
            n269 = local read "Snpx"() -> (w143:refnum<k24>)
            n270 = call "GetWorldPosition.vi"("Snpx"=w143) -> ("UserTool"=→"UserTool":i16, "Cartesian position"=→"Cartesian position":T11, "JointsPosition"=→"JointsPosition":dbl[], "error out"=→"error out":errorcluster)  [unwired: 7 in]
          }
        }
        n271 = case shown="True" w112 {
          frame False {
          }
          frame True {
            n272 = local read "Snpx"() -> (w139:refnum<k24>)
            n273 = call "GetUserFramePosition.vi"("userFrame"="userFrame", "Snpx"=w139) -> ("UserTool"=→"UserTool":i16, "Cartesian position"=→"Cartesian position":T11, "error out"=→"error out 2":errorcluster)  [unwired: 6 in, 1 out]
          }
        }
        n274 = case shown="True" w105 {
          tunnel: "String register" -> [_ w130]
          frame False {
          }
          frame True {
            n275 = local read "Snpx"() -> (w131:refnum<k24>)
            n276 = call "ReadStringRegister.vi"("index"=w130, "Snpx"=w131) -> ("Value"=→"Value":string)  [unwired: 8 in, 1 out]
          }
        }
        n277 = case shown="True" w98 {
          tunnel: "Position register" -> [_ w115]
          tunnel: "Joints position" -> [_ w114]
          frame False {
          }
          frame True {
            n278 = local read "Snpx"() -> (w116:refnum<k24>)
            n279 = call "WriteJointPositionRegister.vi"("Value"=w114, "index"=w115, "Snpx"=w116) -> ()  [unwired: 8 in, 1 out]
          }
        }
        n280 = case shown="True" w103 {
          tunnel: "Position register" -> [_ w124]
          frame False {
          }
          frame True {
            n281 = local read "Snpx"() -> (w125:refnum<k24>)
            n282 = call "ReadPositionRegister.vi"("Snpx"=w125, "index"=w124) -> ("UserFrame"=→"UserFrame":i16, "Cartesian position"=w123:T10, "UserTool"=→"UserTool":i16, "Joint position"=w120:dbl[])  [unwired: 9 in, 1 out]
            n283 = property on="Cartesian position" class="Clust (strict)"("Value"=w123) -> ()  [unwired: 2 in, 2 out]
            n284 = property on="Joints position" class="Arr (strict)"("Value"=w120) -> ()  [unwired: 2 in, 2 out]
          }
        }
        n285 = case shown="True" w104 {
          tunnel: "String register" -> [_ w127]
          tunnel: "New value" -> [_ w126]
          frame False {
          }
          frame True {
            n286 = local read "Snpx"() -> (w128:refnum<k24>)
            n287 = call "WriteStringRegister.vi"("value"=w126, "index"=w127, "Snpx"=w128) -> ()  [unwired: 8 in, 1 out]
          }
        }
        n288 = case shown="True" w111 {
          tunnel: "Numeric register" -> [_ w136]
          frame False {
          }
          frame True {
            n289 = local read "Snpx"() -> (w137:refnum<k24>)
            n290 = call "ReadNumericRegister.vi"("index"=w136, "Snpx"=w137) -> ("Value"=→"Value":sgl)  [unwired: 8 in, 1 out]
          }
        }
        n291 = case shown="True" w102 {
          tunnel: "Cartesian position 2" -> [_ w118]
          tunnel: "Position register" -> [_ w117]
          frame False {
          }
          frame True {
            n292 = local read "Snpx"() -> (w119:refnum<k24>)
            n293 = call "WriteCartesianPositionRegister.vi"("Cartesian position"=w118, "index"=w117, "Snpx"=w119) -> ()  [unwired: 8 in, 1 out]
          }
        }
        n294 = case shown="True" w110 {
          tunnel: "New value" -> [_ w133]
          tunnel: "Numeric register" -> [_ w132]
          frame False {
          }
          frame True {
            n295 = local read "Snpx"() -> (w134:refnum<k24>)
            n296 = call "WriteNumericRegister.vi"("Value"=w133, "index"=w132, "Snpx"=w134) -> ()  [unwired: 8 in, 1 out]
          }
        }
      }
    }
    n297 = property on="SNPX warning" class="Str"("Visible"=w36) -> ()  [unwired: 2 in, 2 out]
    n298 = property on="Read string register" class="Bool"("DisabledEnum"=w24) -> ()  [unwired: 2 in, 2 out]
    n299 = property on="Write string register" class="Bool"("DisabledEnum"=w24) -> ()  [unwired: 2 in, 2 out]
    n300 = property on="Read numeric register" class="Bool"("DisabledEnum"=w24) -> ()  [unwired: 2 in, 2 out]
    n301 = property on="Write numeric register" class="Bool"("DisabledEnum"=w24) -> ()  [unwired: 2 in, 2 out]
    n302 = property on="Write joints position register" class="Bool"("DisabledEnum"=w24) -> ()  [unwired: 2 in, 2 out]
    n303 = property on="Continuous read user frame position" class="Bool (strict)"("DisabledEnum"=w24) -> ()  [unwired: 2 in, 2 out]
    n304 = property on="Write cartesian position register" class="Bool"("DisabledEnum"=w24) -> ()  [unwired: 2 in, 2 out]
    n305 = property on="Continuous read world position" class="Bool (strict)"("DisabledEnum"=w24) -> ()  [unwired: 2 in, 2 out]
    n306 = property on="Read position register" class="Bool"("DisabledEnum"=w24) -> ()  [unwired: 2 in, 2 out]
  }
  "TelnetError" <- "" ("ErrorText")
  "TelnetSucceed" <- FALSE ("Succeed")
  "KclCommand" <- "" ("KclCommand")
  "Telnet warning" <- "Telnet is not connected\nPlease connect to use this panel" ("Telnet warning")
  "FTP warning" <- "FTP is not connected\nPlease connect to use this panel" ("FTP warning")
  "SNPX warning" <- "SNPX is not connected\nPlease connect to use this panel" ("FTP warning")
